vi "Launch ES Actor.vi"(8 "error in":errorcluster, 11 "SCADA in":refnum<class "EMS.lvclass">) -> (0 "error out":errorcluster, 3 "SCADA out":refnum<class "EMS.lvclass">)   [LabVIEW 2018, in "EMS Core.lvlib" / "EMS.lvclass"]
uses:
  EMS.lvclass
  C:/Users/Administrator/Desktop/LabVIEW EMS/EMS Generic Actor/EMS Generic/EMS Generic.lvclass
  C:/Program Files (x86)/National Instruments/LabVIEW 2018/vi.lib/ActorFramework/Actor/Actor.lvclass
  IED Actors/ES Actor/ES/ES.lvclass
  <vilib>/ORNL/CSEISMIC DDS/CSEISMIC DDS Base/Data Types/Controls/DeviceClass Selector.ctl
  EMS.lvclass/EMS.ctl
  <vilib>/ActorFramework/Actor/Actor.lvclass
  <vilib>/ORNL/CSEISMIC DDS/CSEISMIC DDS Base/CSEISMIC DDS.lvclass
  EMS Generic Actor/EMS Generic/EMS Generic.lvclass
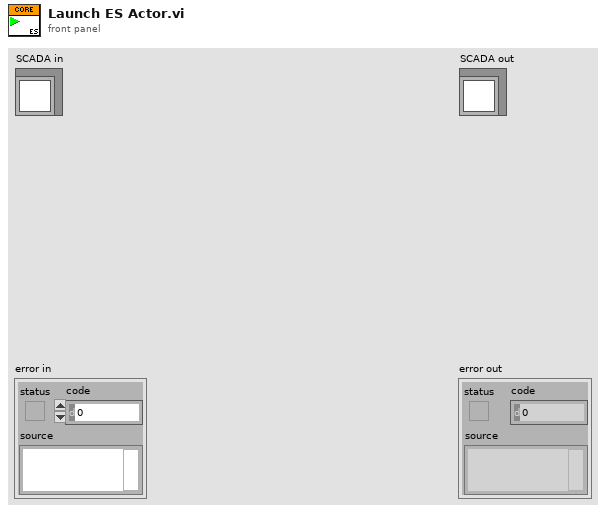
[diagram p1: front panel]
types:
  T1 = typedef "CSEISMIC DDS.lvlib/CSEISMIC DDS.lvclass/DeviceID.ctl" = string
  T2 = typedef "CSEISMIC DDS.lvlib/CSEISMIC DDS.lvclass/DeviceClass Selector.ctl" = u16
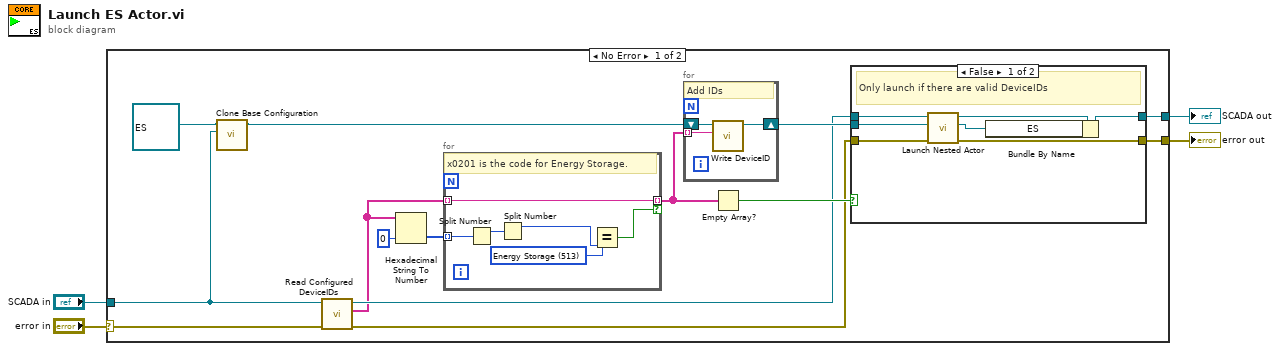
[diagram p0: block diagram]
diagram:
  n1 = case shown="No Error" "error in" {
    selector: "error in" -> [w8 w38]
    tunnel: [w17 w38] -> w3
    tunnel: [w18 w37] -> w1
    tunnel: "SCADA in" -> [w5 w37]
    frame No Error {
      n2 = call-dynamic "Clone Base Configuration.vi"("Source Object"=w5, "Target Object in"=refnum<class "ES.lvclass"> refnum ("ES Actor.lvlib:ES.lvclass")) -> ("Target Object out"=w6:refnum<class "ES.lvclass">)  [unwired: 9 in]
      n3 = call "Read Configured DeviceIDs.vi"("error in"=w8, "EMS Generic in"=w5) -> ("error out"=w12:errorcluster, "DeviceIDs"=w10:T1[], "EMS Generic out"=w13:refnum<class "EMS.lvclass">)  [unwired: 7 in]
      n4 = Hexadecimal String To Number(string=w10, default (0uL)=u64 0 ("default (0 U32)")) -> (number=w9:u64[])  [unwired: 1 in, 1 out]
      n5 = for {
        tunnel: w10 -> [w22] mode=indexing
        tunnel: [w22] -> w15 mode=indexing if=w21
        tunnel: w9 -> [w19] mode=indexing
        w20 = T2 513 items=["Invalid"=0, "IED"=256, "DER"=512, "Relay"=768, "Meter"=1024, "Load"=1280, "Forecast"=1536, "Price"=1792, "Energy Storage"=513, "PV"=514, "Generator"=515, "Smart Relay"=769, "PCC"=770, "Smart Meter"=1025, "PMU"=1026, "HVAC"=1281] ("DeviceClass")
        # "x0201 is the code for Energy Storage."
        n6 = Split Number(x=w19) -> (hi(x)=w24:u32)  [unwired: 1 out]
        n7 = Split Number(x=w24) -> (hi(x)=w23:u16)  [unwired: 1 out]
        n8 = Equal?(x=w23, y=w20) -> (x = y?=w21:bool)
      }
      n9 = for {
        shift-right: [w35] -> w16
        shift-left: w6 -> [w36]
        tunnel: w15 -> [w34] mode=indexing
        # "Add IDs"
        n10 = call-dynamic "Write DeviceID.vi"("DeviceID"=w34, "Device DDS Communications in"=w36) -> ("Device DDS Communications out"=w35:refnum<class "ES.lvclass">)  [unwired: 9 in]
      }
      n11 = Empty Array?(array=w15) -> (empty?=w14:bool)
      n12 = case shown="False" w14 {
        tunnel: [w26 w33] -> w18
        tunnel: w12 -> [w30 w32]
        tunnel: [w29 w32] -> w17
        tunnel: w16 -> [w28 _]
        tunnel: w13 -> [w27 w33]
        frame False {
          # "Only launch if there are valid DeviceIDs"
          n13 = call <vilib>:"Launch Nested Actor.vi"("error in (no error)"=w30, "Nested Actor"=w28, "Caller Actor in"=w27) -> ("error out"=w29:errorcluster, "Nested Actor's Enqueuer"=w25:refnum<class "Message Enqueuer.lvclass">, "Caller Actor out"=w31:refnum<class "EMS.lvclass">)  [unwired: 6 in]
          n14 = Bundle By Name(cluster=w31, "ES"=w25) -> (w26:refnum<class "EMS.lvclass">)
        }
        frame True {
        }
      }
    }
    frame Error {
    }
  }
  "error out" <- w3
  "SCADA out" <- w1
